vi "GVglobalStopFPGA_ECD.vi"() -> ()   [LabVIEW 2017]
panel:
  in  "globalStopFPGA":bool
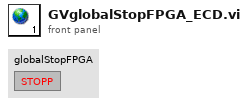
[diagram p1: front panel]
diagram:
